vi "cno_objective function.vi"(7 "function":enum16{"initialize", "execute"}(ring)=enum."execute", 8 "error in (no error)":errorcluster, 10 "user defined functions":T1, 11 "X":dbl[](array[numeric])) -> (0 "error out":errorcluster, 2 "num function calls":i32, 3 "F(X)":dbl[](array[numeric]))   [LabVIEW 2014, in "NI_Gmath.lvlib"]
uses:
  NI_Gmath.lvlib
  cno_user defined functions.ctl
  cno_user objective function ref.ctl
  objective function data.ctl
  cno_output select.ctl
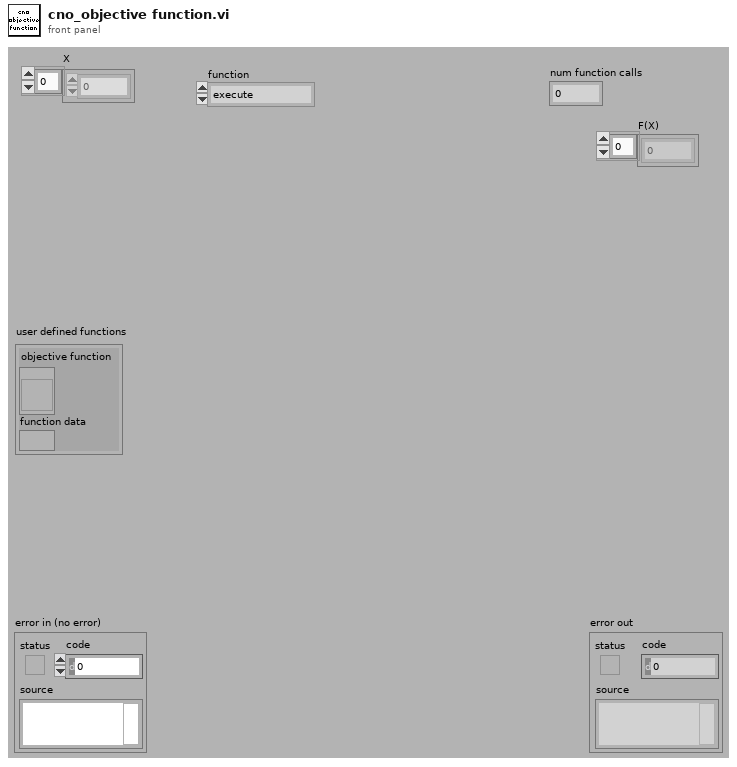
[diagram p1: front panel]
types:
  T1 = typedef "NI_Gmath.lvlib/cno_user defined functions.ctl" = cluster{"objective function":T2, "function data":T3}
  T2 = typedef "NI_Gmath.lvlib/cno_user objective function ref.ctl" = refnum<vi>
  T3 = typedef "NI_Gmath.lvlib/objective function data.ctl" = variant
  T4 = typedef "NI_Gmath.lvlib/cno_output select.ctl" = cluster{"objective function":bool, "equality constraint":bool, "inequality constraint":bool}
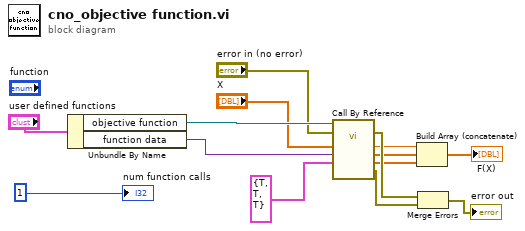
[diagram p0: block diagram]
diagram:
  n1 = Unbundle By Name("user defined functions") -> ("objective function"=w13:T2, "function data"=w2:T3)
  n2 = call-by-ref "?"(reference=w13, error in="error in (no error)", "output selector"=T4 {"objective function"=TRUE, "equality constraint"=TRUE, "inequality constraint"=TRUE}, "function data"=w2, "X"="X") -> (error out=w10:errorcluster, 0:"error out"=w7:errorcluster, "inequality constraint function values"=w6:dbl[], "equality constraint function values"=w5:dbl[], "objective function value"=w4:dbl)  [unwired: 5 in, 1 out]
  n3 = Build Array (concatenate)(w4, w5, w6) -> (→"F(X)":dbl[])
  n4 = Merge Errors(w10, w7) -> (→"error out":errorcluster)
  "num function calls" <- 1
